vi "Max Lines Auto.vi"(8 "error in (no error)":errorcluster, 10 "Camera Setings In":T1={"Exposure Time (ms)"=10.0, "Binning"=enum."2x2", "Scan Mode"=-1, "Frames to Acquire"=1000.0, "Pixel Correction"=FALSE, "Frames to Skip"=0, "File Path"=path "", "Duty cycle"=1.0, "ALEX"=FALSE, "Shutter Enable"=[], "fluidics trigger frame"=0, "Bit Depth"=0, "Image Width (px)"=0, "Image Height (px)"=0, "Horizontal Offset (px)"=0, "Vertical Offset (px)"=0} {"fluidics trigger frame" max=60000 step=1; "Exposure Time (ms)" min=0.1 max=1000.0 step=1.0}, 11 "Hamamatsu Camera in":refnum<class "Hamamatsu Camera.lvclass">) -> (0 "error out":errorcluster, 2 "Camera Settings Out":T1={"Exposure Time (ms)"=100.0, "Binning"=enum."2x2", "Scan Mode"=0, "Frames to Acquire"=1000.0, "Pixel Correction"=FALSE, "Frames to Skip"=0, "File Path"=path "", "Duty cycle"=0.0, "ALEX"=FALSE, "Shutter Enable"=[], "fluidics trigger frame"=0, "Bit Depth"=0, "Image Width (px)"=0, "Image Height (px)"=0, "Horizontal Offset (px)"=0, "Vertical Offset (px)"=0} {"fluidics trigger frame" max=60000 step=1; "Exposure Time (ms)" min=1.0 max=10000.0 step=1.0}, 3 "Hamamatsu Camera out":refnum<class "Hamamatsu Camera.lvclass">, 4 "Allowed scan modes":cluster{"String":string, "Number":i32}[](array[cluster]))   [LabVIEW 2023, in "Hamamatsu Camera.lvlib" / "Hamamatsu Camera.lvclass"]
uses:
  Hamamatsu Camera.lvclass
  Resources/Type Defs/Camera Settings.ctl
  Hamamatsu Camera.lvclass/Hamamatsu Camera.ctl
panel:
  out "Readout Speeds":dbl[](array[numeric])
  out "min read time":dbl
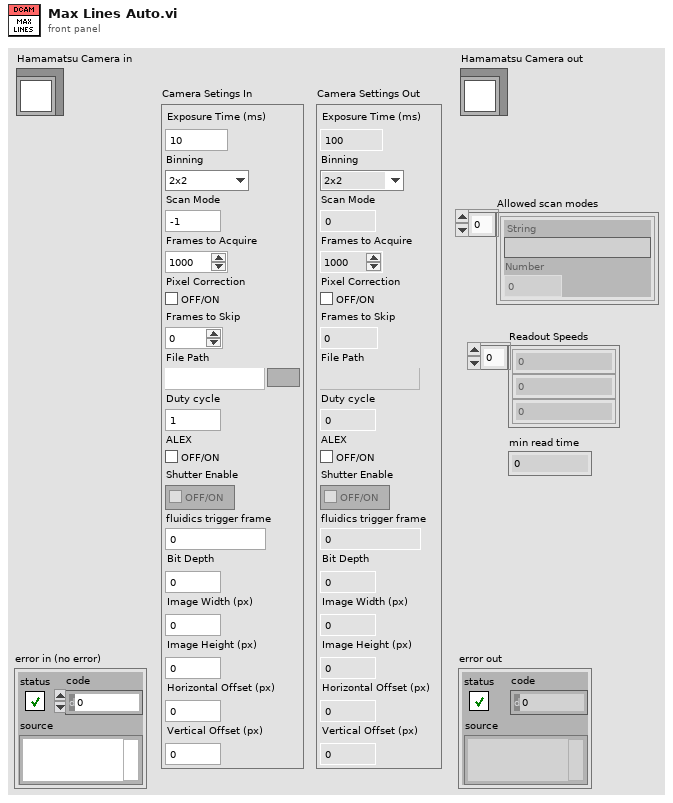
[diagram p1: front panel]
types:
  T1 = typedef "Camera Settings.ctl" = cluster{"Exposure Time (ms)":dbl, "Binning":enum16{"1x1", "2x2", "4x4"}, "Scan Mode":i32, "Frames to Acquire":dbl, "Pixel Correction":bool, "Frames to Skip":u32, "File Path":path, "Duty cycle":dbl, "ALEX":bool, "Shutter Enable":bool[], "fluidics trigger frame":u16, "Bit Depth":u16, "Image Width (px)":u16, "Image Height (px)":u16, "Horizontal Offset (px)":u16, "Vertical Offset (px)":u16}
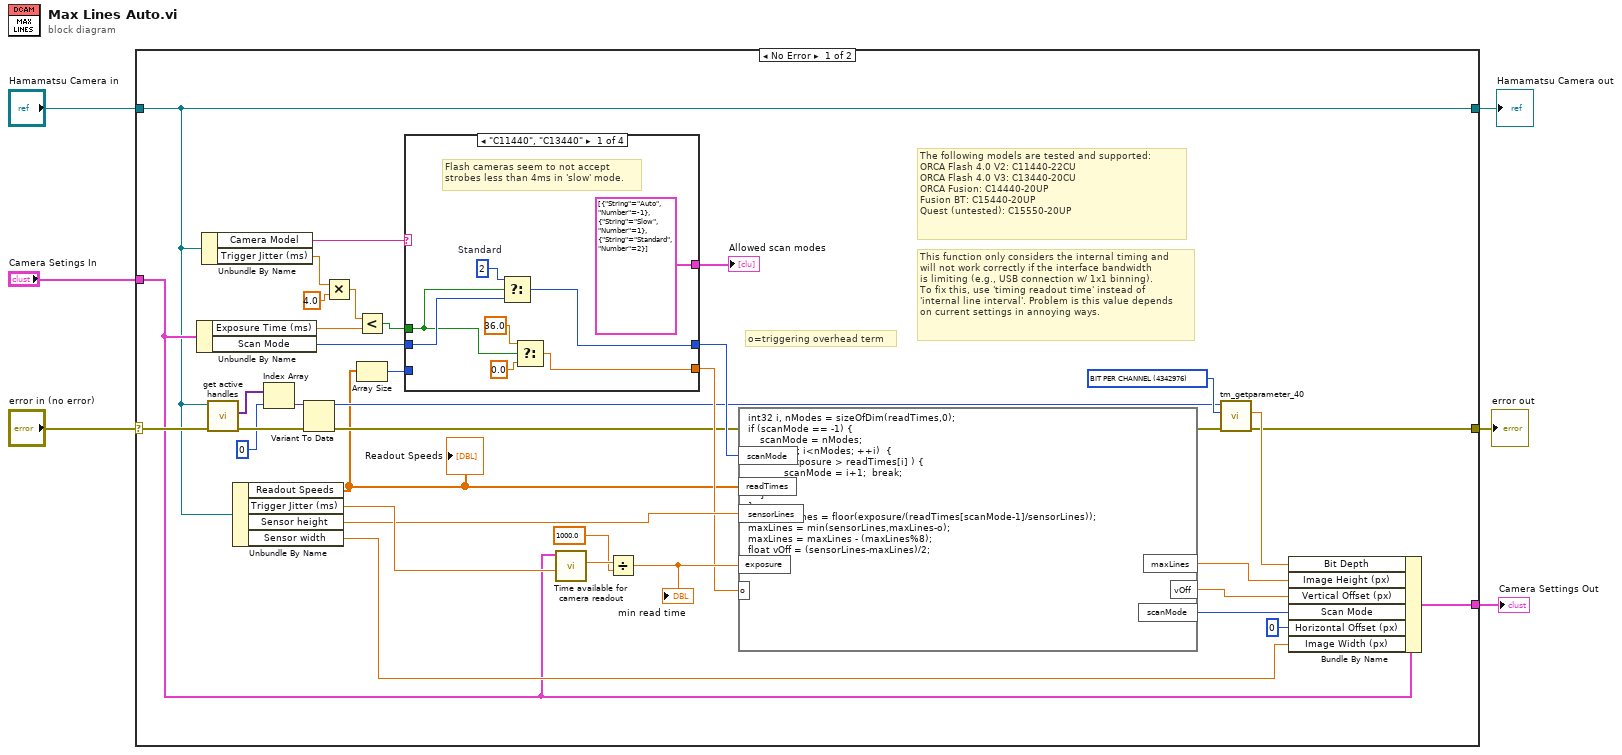
[diagram p0: block diagram]
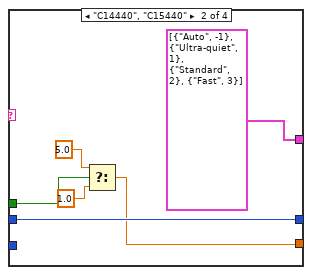
[diagram p2: hidden frame]
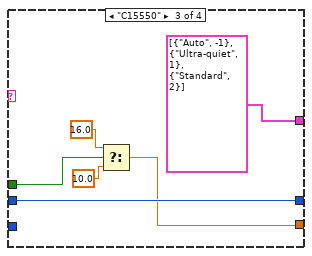
[diagram p3: hidden frame]
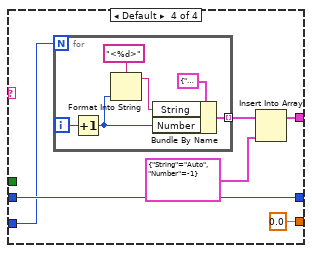
[diagram p4: hidden frame]
diagram:
  n1 = case shown="No Error" "error in (no error)" {
    selector: "error in (no error)" -> [w27 w75]
    tunnel: [w22 w75] -> w5
    tunnel: [w18 w74] -> w3
    tunnel: "Hamamatsu Camera in" -> [w18 w74]
    tunnel: [w26 _] -> w2
    tunnel: "Camera Setings In" -> [w19 _]
    frame No Error {
      w40 = u32 4342976 items=["SENSOR MODE"=4212128, "READOUT SPEED"=4211872, "READOUT DIRECTION"=4211904, "BIT PER CHANNEL"=4342976, "TRIGGER SOURCE"=1066144, "TRIGGER MODE"=1066400, "TRIGGER ACTIVE"=1066160, "TRIGGER GLOBAL EXPOSURE"=2049680, "TRIGGER POLARITY"=1066416, "TRIGGER CONNECTOR"=1066432, "TRIGGER DELAY"=1066480, "SENSOR TEMPERATURE"=2115232, "SENSOR COOLER STATUS"=2115280, "EXPOSURE TIME"=2049184, "DEFECT CORRECT MODE"=4670368, "HOT PIXEL CORRECT LEVEL"=4670400, "BINNING"=4215968, "TIMING READOUT TIME"=4223904, "INTERNAL FRAME RATE"=4225952, "INTERNAL FRAME INTERVAL"=4225968, "INTERNAL LINE SPEED"=4226000, "INTERNAL LINE INTERVAL"=4226016, "IMAGE WIDTH"=4343200, "IMAGE HEIGHT"=4343216, "IMAGE ROWBYTES"=4343232, "IMAGE FRAMEBYTES"=4343248, "IMAGE PIXEL TYPE"=4343296, "NUMBER OF OUTPUT TRIGGER CONNECTOR"=1852320, "OUTPUT TRIGGER SOURCE[0]"=1852576, "OUTPUT TRIGGER SOURCE[1]"=1852832, "OUTPUT TRIGGER SOURCE[2]"=1853088, "OUTPUT TRIGGER POLARITY[0]"=1852592, "OUTPUT TRIGGER POLARITY[1]"=1852848, "OUTPUT TRIGGER POLARITY[2]"=1853104, "OUTPUT TRIGGER ACTIVE[0]"=1852608, "OUTPUT TRIGGER ACTIVE[1]"=1852864, "OUTPUT TRIGGER ACTIVE[2]"=1853120, "OUTPUT TRIGGER DELAY[0]"=1852624, "OUTPUT TRIGGER DELAY[1]"=1852880, "OUTPUT TRIGGER DELAY[2]"=1853136, "OUTPUT TRIGGER PERIOD[0]"=1852640, "OUTPUT TRIGGER PERIOD[1]"=1852896, "OUTPUT TRIGGER PERIOD[2]"=1853152, "OUTPUT TRIGGER KIND[0]"=1852656, "OUTPUT TRIGGER KIND[1]"=1852912, "OUTPUT TRIGGER KIND[2]"=1853168, "OUTPUT TRIGGER PRE HSYNC COUNT"=1852704] ("Parameter")
      # "This function only considers the internal timing and\nwill not work correctly if the interface bandwidth\nis limiting (e.g., USB connection w/ 1x1 binning).\nTo fix this, use 'timing readout time' instead of\n'internal line interval'. Problem is this value depends\non current settings in annoying ways."
      # "o=triggering overhead term"
      # "The following models are tested and supported:\nORCA Flash 4.0 V2: C11440-22CU\nORCA Flash 4.0 V3: C13440-20CU\nORCA Fusion: C14440-20UP\nFusion BT: C15440-20UP\nQuest (untested): C15550-20UP"
      n2 = Unbundle By Name(w19) -> ("Exposure Time (ms)"=w11:dbl, "Scan Mode"=w31:i32)
      n3 = Unbundle By Name(w18) -> ("Camera Model"=w17:string, "Trigger Jitter (ms)"=w8:dbl)
      n4 = call-dynamic "get active handles.vi"("error in (no error)"=w27, "Camera in"=w18) -> ("error out"=w28:errorcluster, "Handles"=w25:variant[])  [unwired: 5 in, 3 out]
      n5 = Unbundle By Name(w18) -> ("Readout Speeds"=w13:dbl[], "Trigger Jitter (ms)"=w29:dbl, "Sensor height"=w20:dbl, "Sensor width"=w21:dbl)
      "Readout Speeds" <- w13
      n6 = Index Array(array=w25, index=0) -> (element=w24:variant)
      n7 = Variant To Data(error in=w28, Variant=w24) -> (data=w15:u32, error out=w14:errorcluster)  [unwired: 1 in]
      n8 = Multiply(x=w8, y=4.0) -> (x*y=w9:dbl)
      n9 = Less?(x=w9, y=w11) -> (x < y?=w10:bool)
      n10 = Array Size(array=w13) -> (size(s)=w12:i32)
      n11 = case shown="\"C11440\", \"C13440\"" w17 {
        tunnel: [cluster{"String":string, "Number":i32}[] [{"String"="Auto", "Number"=-1}, {"String"="Slow", "Number"=1}, {"String"="Standard", "Number"=2}] cluster{"String":string, "Number":i32}[] [{"String"="Auto", "Number"=-1}, {"String"="Ultra-quiet", "Number"=1}, {"String"="Standard", "Number"=2}, {"String"="Fast", "Number"=3}] cluster{"String":string, "Number":i32}[] [{"String"="Auto", "Number"=-1}, {"String"="Ultra-quiet", "Number"=1}, {"String"="Standard", "Number"=2}] w65] -> w41
        tunnel: w10 -> [w42 w50 w56 _]
        tunnel: w31 -> [w48 w54 w60 w67]
        tunnel: [w47 w54 w60 w67] -> w30
        tunnel: w12 -> [_ _ _ w66]
        tunnel: [w43 w51 w57 0.0] -> w16
        frame "C11440", "C13440" {
          w46 = 2  # Standard
          # "Flash cameras seem to not accept \nstrobes less than 4ms in 'slow' mode."
          n12 = Select(t=w46, s=w42, f=w48) -> (s? t:f=w47:i32)
          n13 = Select(t=36.0, s=w42, f=0.0) -> (s? t:f=w43:dbl)
        }
        frame "C14440", "C15440" {
          n14 = Select(t=5.0, s=w50, f=1.0) -> (s? t:f=w51:dbl)
        }
        frame "C15550" {
          n15 = Select(t=16.0, s=w56, f=10.0) -> (s? t:f=w57:dbl)
        }
        frame Default {
          n16 = for {
            N: w66 -> [_]
            tunnel: [w73] -> w64 mode=indexing
            i -> [w72]
            n17 = Increment(x=w72) -> (x+1=w70:i32)
            n18 = Format Into String(format string="<%d>", w70) -> (resulting string=w71:string)  [unwired: 2 in, 1 out]
            n19 = Bundle By Name(cluster=cluster{"String":string, "Number":i32} {"String"="Auto", "Number"=-1}, "String"=w71, "Number"=w70) -> (w73:cluster{"String":string, "Number":i32})
          }
          n20 = Insert Into Array(array=w64, new element=cluster{"String":string, "Number":i32} {"String"="Auto", "Number"=-1}) -> (w65:cluster{"String":string, "Number":i32}[])  [unwired: 1 in]
        }
      }
      "Allowed scan modes" <- w41
      n21 = call "Time available for camera readout.vi"("Trigger Jitter (ms)"=w29, "Camera Settings"=w19) -> ("Min readout time (ms)"=w35:dbl)  [unwired: 8 in, 1 out]
      n22 = Divide(x=w35, y=1000.0) -> (x/y=w33:dbl)
      "min read time" <- w33
      n23 = formula code="int32 i, nModes = sizeOfDim(readTimes,0);\nif (scanMode == -1) {\n    scanMode = nModes;\n    for (i=0; i<nModes; ++i)  {\n        if ( exposure > readTimes[i] ) {\n            scanMode = i+1;  break;\n        }\n    }\n}\nfloat maxLines = floor(exposure/(readTimes[scanMode-1]/sensorLines));\nmaxLines = min(sensorLines,maxLines-o);\nmaxLines = maxLines - (maxLines%8);\nfloat vOff = (sensorLines-maxLines)/2;"("readTimes"=w13, "sensorLines"=w20, "exposure"=w33, "scanMode"=w30, "o"=w16) -> ("maxLines"=w38:dbl, "vOff"=w37:dbl, "scanMode"=w32:i32)
      n24 = call <userlib>:"tm_getparameter_40.vi"("error in (no error)"=w14, "Parameter"=w40, "Handle in"=w15) -> ("error out"=w22:errorcluster, "Value out"=w39:dbl)  [unwired: 6 in, 1 out]
      n25 = Bundle By Name(cluster=w19, "Bit Depth"=w39, "Image Height (px)"=w38, "Vertical Offset (px)"=w37, "Scan Mode"=w32, "Horizontal Offset (px)"=u16 0, "Image Width (px)"=w21) -> (w26:T1)
    }
    frame Error {
    }
  }
  "error out" <- w5
  "Hamamatsu Camera out" <- w3
  "Camera Settings Out" <- w2
